vi "sandbox.vi"() -> ()   [LabVIEW 2019, in "ModbusSp.lvclass"]
uses:
  ModbusSp.lvclass
  WriteData.ctl
  ReadData.ctl
  STS REG.ctl
  CMD REG.ctl
  <vilib>/NI/Modbus Library/Network Protocol/Network Slave/TCP/Connection.ctl
  ModbusSp.lvclass/ModbusSp.ctl
  ConvertWriteDataToReg.vi
  ConvertRegToReadData.vi
  Clear CMD Reg.vi
  Modbus Data Type Conversation/SGL Array to U16 Array.vi
  Modbus Data Type Conversation/U16 Array TO SGL Array.vi
  Modbus Data Type Conversation/SGL to U16.vi
  <vilib>/NI/Modbus Library/API/Slave/Modbus Slave.lvclass
  <vilib>/NI/Modbus Library/Network Protocol/Network Slave/TCP/TCP Slave.lvclass
panel:
  out "TCP Connection Count":u32
  out "TCP Connection List":T1[](array[typedef])
  out "Waveform Chart 2":sgl(graph)
  out "Waveform Chart":sgl(graph)
  out "CMD REG":T2
  in  "STS REG":T3
  out "size(s)":i32
  out "register readed":u16[](array[numeric])
  out "registers to write":u16[](array[numeric])
  out "Data Read":T4
  in  "Data Write":T5
  in  "stop":bool
  out "error out":errorcluster
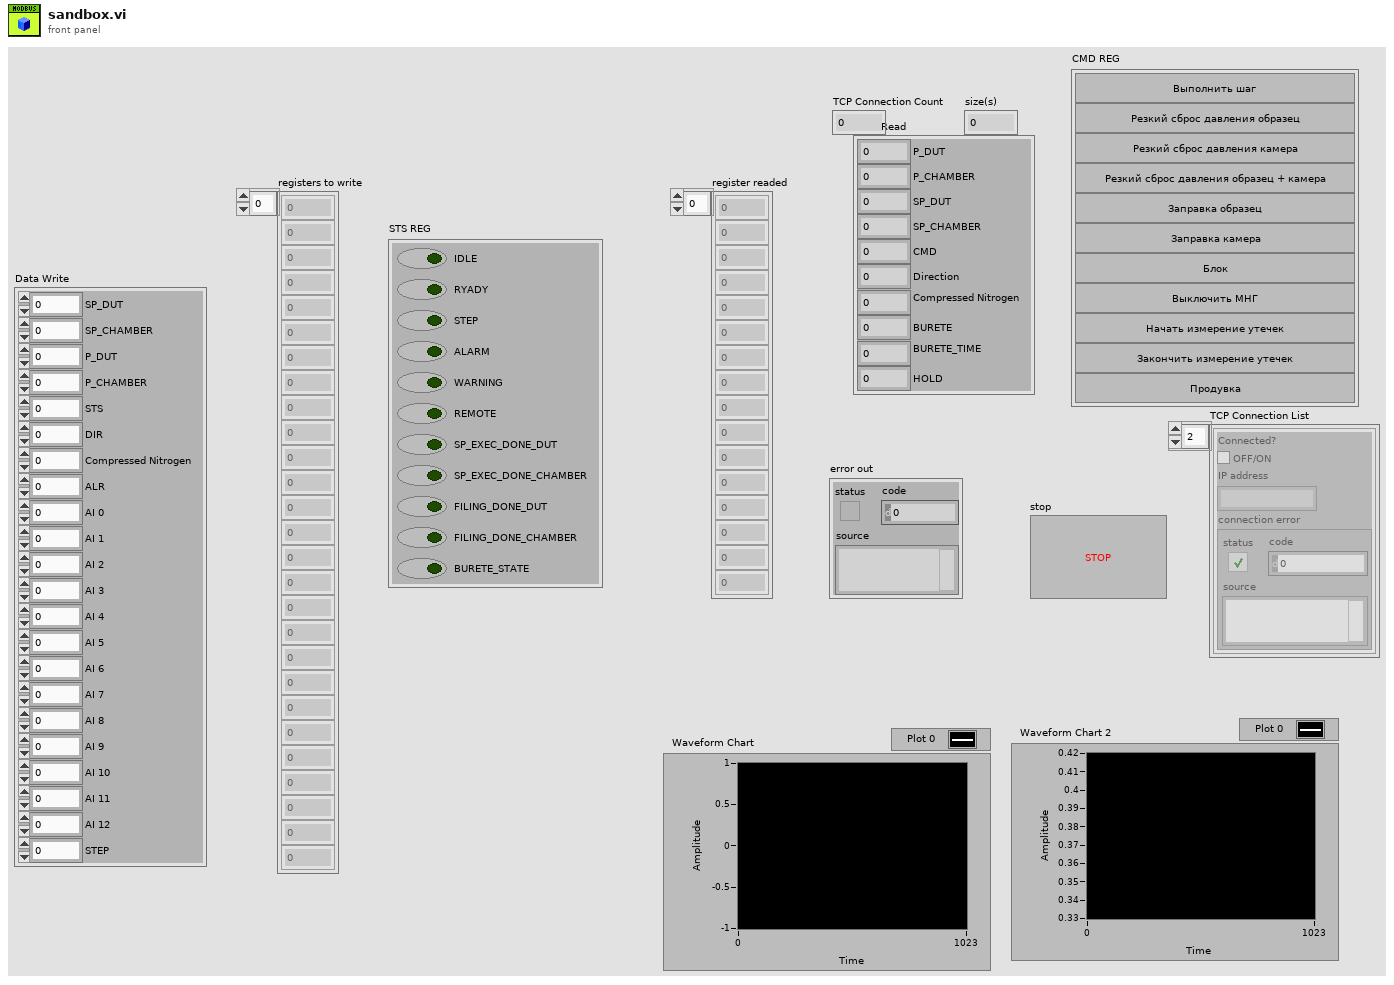
[diagram p1: front panel]
types:
  T1 = typedef "TCP Slave.lvclass/Connection.ctl" = cluster{"Connected?":bool, "IP address":string, "connection error":errorcluster}
  T2 = typedef "CMD REG.ctl" = cluster{"EXECUTE_SP":bool, "ALARM_PRESS_DOWN_DUT":bool, "ALARM_PRESS_DOWN_CHAMBER":bool, "ALARM_PRESS_DOWN_DUT_CHAMBER":bool, "FILING_DUT":bool, "FILING_CHAMBER":bool, "BLOCK":bool, "PUMP_STATION_OFF":bool, "Leak start":bool, "Leak stop":bool, "Drain":bool}
  T3 = typedef "STS REG.ctl" = cluster{"IDLE":bool, "RYADY":bool, "STEP":bool, "ALARM":bool, "WARNING":bool, "REMOTE":bool, "SP_EXEC_DONE_DUT":bool, "SP_EXEC_DONE_CHAMBER":bool, "FILING_DONE_DUT":bool, "FILING_DONE_CHAMBER":bool, "BURETE_STATE":bool}
  T4 = typedef "ModbusSp.lvclass/ReadData.ctl" = cluster{"P_DUT":sgl, "P_CHAMBER":sgl, "SP_DUT":sgl, "SP_CHAMBER":sgl, "CMD":u16, "Direction":u16, "Compressed Nitrogen":u16, "BURETE":u16, "BURETE_TIME":u16, "HOLD":u16}
  T5 = typedef "ModbusSp.lvclass/WriteData.ctl" = cluster{"SP_DUT":sgl, "SP_CHAMBER":sgl, "P_DUT":sgl, "P_CHAMBER":sgl, "STS":u16, "DIR":u16, "Compressed Nitrogen":u16, "ALR":u16, "AI 0":sgl, "AI 1":sgl, "AI 2":sgl, "AI 3":sgl, "AI 4":sgl, "AI 5":sgl, "AI 6":sgl, "AI 7":sgl, "AI 8":sgl, "AI 9":sgl, "AI 10":sgl, "AI 11":sgl, "AI 12":sgl, "STEP":u16}
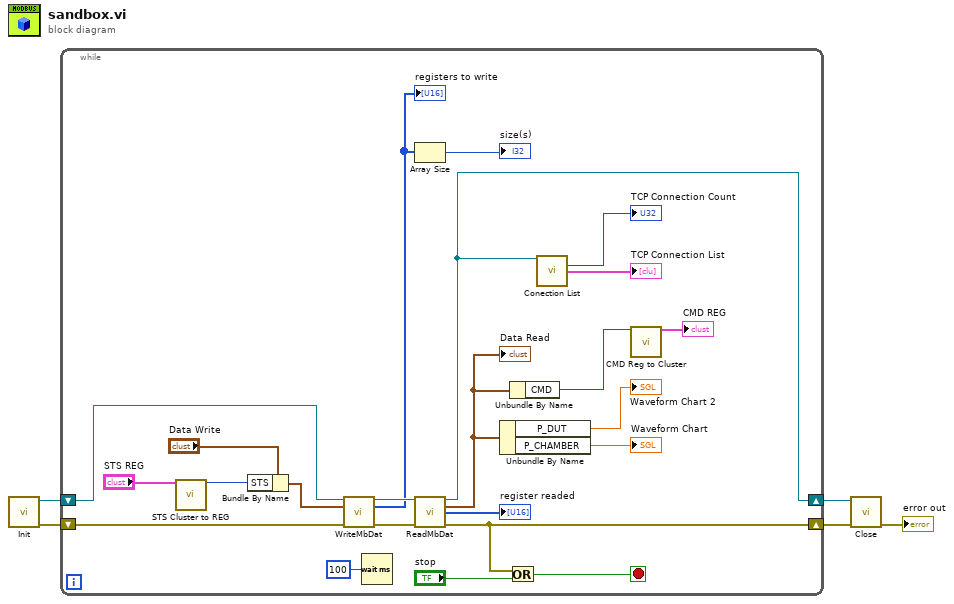
[diagram p0: block diagram]
diagram:
  n1 = call "Init.vi"() -> ("error out"=w4:errorcluster, "ModbusSp out"=w5:refnum<class "ModbusSp.lvclass">)  [unwired: 10 in]
  n2 = while {
    shift-right: [w8] -> w2
    shift-left: w5 -> [w28]
    shift-right: [w21] -> w3
    shift-left: w4 -> [w27]
    stop <- w22 stop-if-true
    n3 = call "STS Cluster to REG.vi"("STS REG"="STS REG") -> ("U16"=w15:u16)  [unwired: 14 in]
    n4 = Bundle By Name(cluster="Data Write", "STS"=w15) -> (w16:T5)
    n5 = call "WriteMbDat.vi"("ModbusSp in"=w28, "Data Write"=w16, "error in (no error)"=w27) -> ("ModbusSp out"=w26:refnum<class "ModbusSp.lvclass">, "registers to write"=w18:u16[], "error out"=w25:errorcluster)  [unwired: 10 in]
    "registers to write" <- w18
    n6 = Wait (ms)(milliseconds to wait=u32 100) -> ()  [unwired: 1 out]
    n7 = Array Size(array=w18) -> (size(s)=→"size(s)":i32)
    n8 = call "ReadMbDat.vi"("ModbusSp in"=w26, "error in (no error)"=w25) -> ("ModbusSp out"=w8:refnum<class "ModbusSp.lvclass">, "Data Read"=w11:T4, "register readed"=→"register readed":u16[], "error out"=w21:errorcluster)  [unwired: 10 in]
    "Data Read" <- w11
    n9 = Unbundle By Name(w11) -> ("P_DUT"=→"Waveform Chart 2":sgl, "P_CHAMBER"=→"Waveform Chart":sgl)
    n10 = Or(x=w21, y="stop") -> (x .or. y?=w22:bool)
    n11 = Unbundle By Name(w11) -> ("CMD"=w13:u16)
    n12 = call "Conection List.vi"("ModbusSp in"=w8) -> ("TCP Connection Count"=→"TCP Connection Count":u32, "TCP Connection List"=→"TCP Connection List":T1[])  [unwired: 11 in, 2 out]
    n13 = call "CMD Reg to Cluster.vi"("CMD Reg"=w13) -> ("CMD REG"=→"CMD REG":T2)  [unwired: 14 in]
  }
  n14 = call "Close.vi"("error in (no error)"=w3, "ModbusSp in"=w2) -> ("error out"=→"error out":errorcluster)  [unwired: 8 in, 1 out]
